vi "Write Return FIFO.vi"(8 "error in (no error)":errorcluster, 9 "timeout in ms (0)":i32 format="%d ms", 11 "Transfer Group in":refnum<class "Transfer Group.lvclass">) -> (0 "error out":errorcluster, 1 "timed out?":bool, 3 "Transfer Group out":refnum<class "Transfer Group.lvclass">)   [LabVIEW 2017, in "DSF Core.lvlib" / "Transfer Group.lvclass"]
uses:
  Transfer Group.lvclass
  Transfer Group.lvclass/Transfer Group.ctl
  Timing/Timing.lvclass/Timing.ctl
  Timing/Timing.lvclass
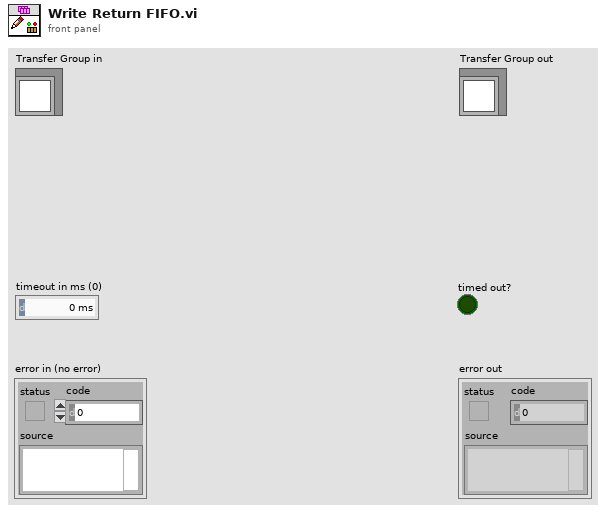
[diagram p1: front panel]
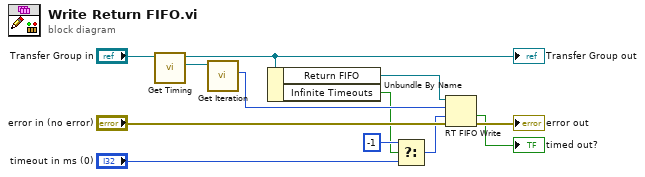
[diagram p0: block diagram]
diagram:
  n1 = call "Get Timing.vi"("Transfer Group in"="Transfer Group in") -> ("Timing"=w9:refnum<class "Timing.lvclass">, "Transfer Group out"=w7:refnum<class "Transfer Group.lvclass">)  [unwired: 9 in]
  "Transfer Group out" <- w7
  n2 = call "Get Iteration.vi"("Timing in"=w9) -> ("Iteration"=w3:u64)  [unwired: 9 in, 1 out]
  n3 = Unbundle By Name(w7) -> ("Return FIFO"=w1:refnum<k33>, "Infinite Timeouts"=w2:bool)
  n4 = Select(t=-1, s=w2, f="timeout in ms (0)") -> (s? t:f=w4:i32)
  n5 = RT FIFO Write(0:w1, 1:w3, 2:w4, 3:"error in (no error)") -> (10:→"timed out?":bool, 11:→"error out":errorcluster)  [unwired: 1 in, 2 out]
